vi "phase.vi"() -> ()   [LabVIEW 2020]
uses:
  <vilib>/measure/NI_MABase.lvlib
panel:
  in  "alharmonikus":dbl=2.0 format="%#_13g"
  in  "felharmonikus":dbl=14.0 format="%#_13g"
  out "Waveform Graph":waveform(dbl)(graph)
  out "PSD":cluster{"f0":dbl, "df":dbl, "magnitude":dbl[]}(graph)
  out "max value":dbl
  out "freq":dbl
  out "Csapásszám [stroke/m]":dbl
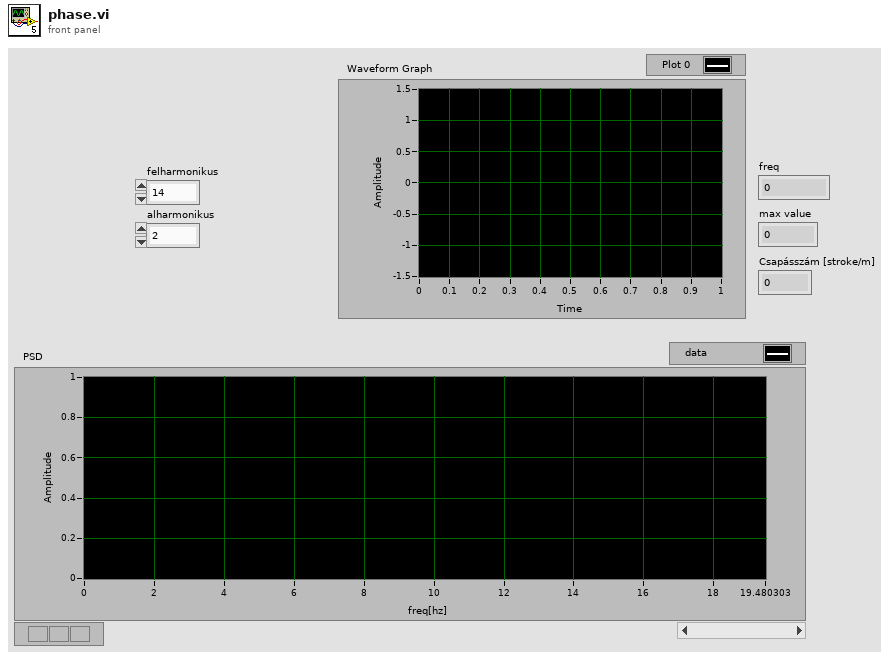
[diagram p1: front panel]
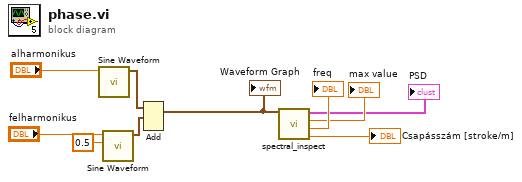
[diagram p0: block diagram]
diagram:
  n1 = call <vilib>:"Sine Waveform.vi"("frequency"="alharmonikus") -> ("signal out"=w6:waveform(dbl))  [unwired: 9 in, 1 out]
  n2 = call <vilib>:"Sine Waveform.vi"("amplitude"=0.5, "frequency"="felharmonikus") -> ("signal out"=w1:waveform(dbl))  [unwired: 8 in, 1 out]
  n3 = Add(1:w1, 2:w6) -> (0:w2:waveform(dbl))  [unwired: 1 in, 1 out]
  "Waveform Graph" <- w2
  n4 = call "spectral_inspect.vi"("waveform"=w2) -> ("Csapásszám [stroke/min]"=→"Csapásszám [stroke/m]":dbl, "freq"=→"freq":dbl, "amplitude"=→"max value":dbl, "PSD"=→"PSD":cluster{"f0":dbl, "df":dbl, "magnitude":dbl[]})  [unwired: 6 in, 1 out]
